vi "Test Tokenizer Number Recognition.vi"(8 "error in (no error)":errorcluster) -> (0 "error out":errorcluster)   [LabVIEW 2019]
uses:
  PathTokenizer/PathTokenizer.lvclass
  PathTokenizer/PathTokenizer.lvclass/PathTokenizer.ctl
  <vilib>/addons/_JKI Toolkits/Caraya/classes/Assert/Assert Equal Value_Variant.vi
  <vilib>/addons/_JKI Toolkits/Caraya/classes/Assert/Assert Error.vi
  <vilib>/addons/_JKI Toolkits/Caraya/classes/Test/Test.lvclass
  <vilib>/addons/_JKI Toolkits/Caraya/classes/Assert/Assert.lvclass
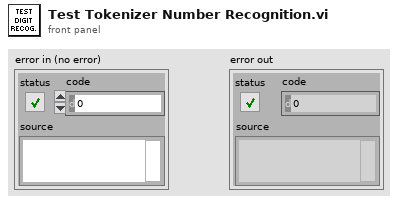
[diagram p1: front panel]
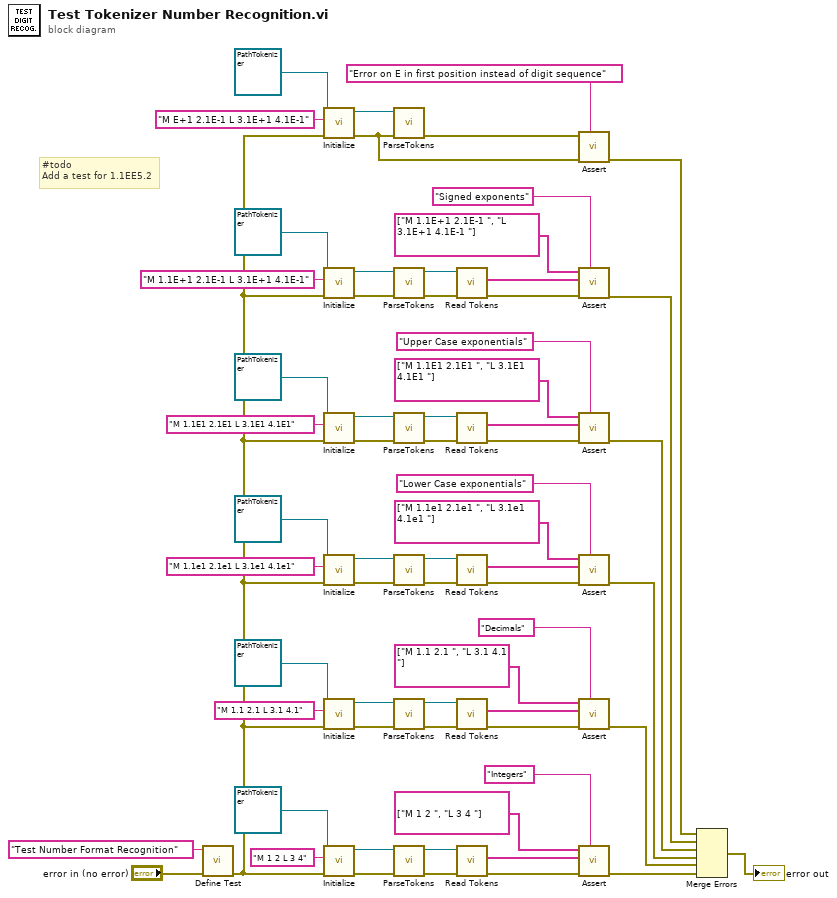
[diagram p0: block diagram]
diagram:
  # "#todo\nAdd a test for 1.1EE5.2"
  n1 = call <vilib>:"Define Test.vi"("error in (no error)"="error in (no error)", "Label (VI Title)"="Test Number Format Recognition") -> ("error out"=w1:errorcluster)  [unwired: 8 in, 1 out]
  n2 = call "Initialize.vi"("error in (no error)"=w1, "Path Command Text"="M E+1 2.1E-1 L 3.1E+1 4.1E-1", "PathTokenizer in"=refnum<class "PathTokenizer.lvclass"> refnum) -> ("error out"=w4:errorcluster, "PathTokenizer out"=w5:refnum<class "PathTokenizer.lvclass">)  [unwired: 7 in]
  n3 = call "Initialize.vi"("error in (no error)"=w1, "Path Command Text"="M 1.1E+1 2.1E-1 L 3.1E+1 4.1E-1", "PathTokenizer in"=refnum<class "PathTokenizer.lvclass"> refnum) -> ("error out"=w18:errorcluster, "PathTokenizer out"=w19:refnum<class "PathTokenizer.lvclass">)  [unwired: 7 in]
  n4 = call "Initialize.vi"("error in (no error)"=w1, "Path Command Text"="M 1.1E1 2.1E1 L 3.1E1 4.1E1", "PathTokenizer in"=refnum<class "PathTokenizer.lvclass"> refnum) -> ("error out"=w22:errorcluster, "PathTokenizer out"=w21:refnum<class "PathTokenizer.lvclass">)  [unwired: 7 in]
  n5 = call "Initialize.vi"("error in (no error)"=w1, "Path Command Text"="M 1.1e1 2.1e1 L 3.1e1 4.1e1", "PathTokenizer in"=refnum<class "PathTokenizer.lvclass"> refnum) -> ("error out"=w40:errorcluster, "PathTokenizer out"=w41:refnum<class "PathTokenizer.lvclass">)  [unwired: 7 in]
  n6 = call "Initialize.vi"("error in (no error)"=w1, "Path Command Text"="M 1.1 2.1 L 3.1 4.1", "PathTokenizer in"=refnum<class "PathTokenizer.lvclass"> refnum) -> ("error out"=w44:errorcluster, "PathTokenizer out"=w43:refnum<class "PathTokenizer.lvclass">)  [unwired: 7 in]
  n7 = call "Initialize.vi"("error in (no error)"=w1, "Path Command Text"="M 1 2 L 3 4", "PathTokenizer in"=refnum<class "PathTokenizer.lvclass"> refnum) -> ("error out"=w62:errorcluster, "PathTokenizer out"=w63:refnum<class "PathTokenizer.lvclass">)  [unwired: 7 in]
  n8 = call "ParseTokens.vi"("error in (no error)"=w4, "PathTokenizer in"=w5) -> ("error out"=w3:errorcluster)  [unwired: 8 in, 1 out]
  n9 = call "ParseTokens.vi"("error in (no error)"=w18, "PathTokenizer in"=w19) -> ("error out"=w16:errorcluster, "PathTokenizer out"=w17:refnum<class "PathTokenizer.lvclass">)  [unwired: 8 in]
  n10 = call "ParseTokens.vi"("error in (no error)"=w22, "PathTokenizer in"=w21) -> ("error out"=w24:errorcluster, "PathTokenizer out"=w23:refnum<class "PathTokenizer.lvclass">)  [unwired: 8 in]
  n11 = call "ParseTokens.vi"("error in (no error)"=w40, "PathTokenizer in"=w41) -> ("error out"=w38:errorcluster, "PathTokenizer out"=w39:refnum<class "PathTokenizer.lvclass">)  [unwired: 8 in]
  n12 = call "ParseTokens.vi"("error in (no error)"=w44, "PathTokenizer in"=w43) -> ("error out"=w46:errorcluster, "PathTokenizer out"=w45:refnum<class "PathTokenizer.lvclass">)  [unwired: 8 in]
  n13 = call "ParseTokens.vi"("error in (no error)"=w62, "PathTokenizer in"=w63) -> ("error out"=w60:errorcluster, "PathTokenizer out"=w61:refnum<class "PathTokenizer.lvclass">)  [unwired: 8 in]
  n14 = call "Read Tokens.vi"("error in (no error)"=w16, "PathTokenizer in"=w17) -> ("error out"=w15:errorcluster, "Tokens"=w12:string[])  [unwired: 7 in, 1 out]
  n15 = call "Read Tokens.vi"("error in (no error)"=w24, "PathTokenizer in"=w23) -> ("error out"=w25:errorcluster, "Tokens"=w28:string[])  [unwired: 7 in, 1 out]
  n16 = call "Read Tokens.vi"("error in (no error)"=w38, "PathTokenizer in"=w39) -> ("error out"=w37:errorcluster, "Tokens"=w34:string[])  [unwired: 7 in, 1 out]
  n17 = call "Read Tokens.vi"("error in (no error)"=w46, "PathTokenizer in"=w45) -> ("error out"=w47:errorcluster, "Tokens"=w50:string[])  [unwired: 7 in, 1 out]
  n18 = call "Read Tokens.vi"("error in (no error)"=w60, "PathTokenizer in"=w61) -> ("error out"=w59:errorcluster, "Tokens"=w55:string[])  [unwired: 7 in, 1 out]
  n19 = call-poly <vilib>:"Assert.vi"("Label"="Error on E in first position instead of digit sequence", "error in (no error)"=w4, "Error?"=w3) -> ("error out"=w2:errorcluster)  [unwired: 7 in, 1 out]
  n20 = call-poly <vilib>:"Assert.vi"("Label"="Signed exponents", "error in (no error)"=w15, "Y"=w12, "X"=string[] ["M 1.1E+1 2.1E-1 ", "L 3.1E+1 4.1E-1 "] ("Tokens")) -> ("error out"=w9:errorcluster)  [unwired: 6 in, 1 out]
  n21 = call-poly <vilib>:"Assert.vi"("Label"="Upper Case exponentials", "error in (no error)"=w25, "Y"=w28, "X"=string[] ["M 1.1E1 2.1E1 ", "L 3.1E1 4.1E1 "] ("Tokens")) -> ("error out"=w20:errorcluster)  [unwired: 6 in, 1 out]
  n22 = call-poly <vilib>:"Assert.vi"("Label"="Lower Case exponentials", "error in (no error)"=w37, "Y"=w34, "X"=string[] ["M 1.1e1 2.1e1 ", "L 3.1e1 4.1e1 "] ("Tokens")) -> ("error out"=w32:errorcluster)  [unwired: 6 in, 1 out]
  n23 = call-poly <vilib>:"Assert.vi"("Label"="Decimals", "error in (no error)"=w47, "Y"=w50, "X"=string[] ["M 1.1 2.1 ", "L 3.1 4.1 "] ("Tokens")) -> ("error out"=w42:errorcluster)  [unwired: 6 in, 1 out]
  n24 = call-poly <vilib>:"Assert.vi"("Label"="Integers", "error in (no error)"=w59, "Y"=w55, "X"=string[] ["M 1 2 ", "L 3 4 "] ("Tokens")) -> ("error out"=w56:errorcluster)  [unwired: 6 in, 1 out]
  n25 = Merge Errors(w2, w9, w20, w32, w42, w56) -> (→"error out":errorcluster)
